vi "StageControl.vi"(9 "Stage Serial Number":i32=94839332, 11 "MG17Motor":refnum<k7>(container)) -> (0 "error IO":errorcluster, 3 "reference out":refnum<k7>)   [LabVIEW 2012]
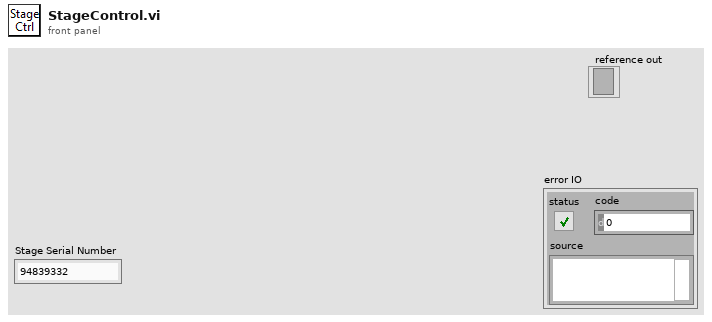
[diagram p1: front panel]
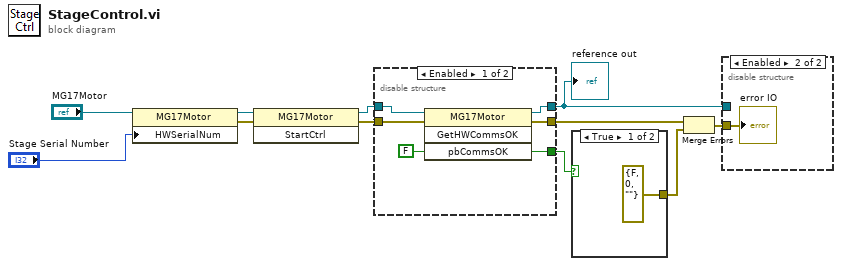
[diagram p0: block diagram]
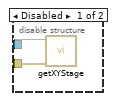
[diagram p2: hidden frame]
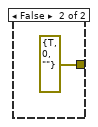
[diagram p4: hidden frame]
diagram:
  n1 = property class="MG17Motor"(reference="MG17Motor", "HWSerialNum"="Stage Serial Number") -> (reference out=w9:refnum<k7>, error out=w5:errorcluster)  [unwired: 1 in]
  n2 = invoke class="MG17Motor" method="StartCtrl"(reference=w9, error in=w5) -> (reference out=w11:refnum<k7>, error out=w10:errorcluster)  [unwired: 1 in, 1 out]
  n3 = disable-structure shown="Enabled" {
    disable-tunnel: w11 -> [w17 w19]
    disable-tunnel: w10 -> [w16 w18]
    disable-tunnel: [w14 _] -> w8
    disable-tunnel: [w13 w18] -> w7
    disable-tunnel: [w12 w19] -> w4
    frame Enabled {
      n4 = invoke class="MG17Motor" method="GetHWCommsOK"(reference=w17, error in=w16, "pbCommsOK"=FALSE) -> (reference out=w12:refnum<k7>, error out=w13:errorcluster, "pbCommsOK"=w14:bool)  [unwired: 1 in, 1 out]
    }
    frame Disabled {
    }
  }
  "reference out" <- w4
  n5 = case shown="True" w8 {
    tunnel: [errorcluster {"status"=FALSE, "code"=0, "source"=""} ("error in (no error)") errorcluster {"status"=TRUE, "code"=0, "source"=""} ("error in (no error)")] -> w6
    frame True {
    }
    frame False {
    }
  }
  n6 = Merge Errors(w7, w6) -> (w1:errorcluster)
  n7 = disable-structure shown="Enabled" {
    disable-tunnel: w4 -> [w23 _]
    disable-tunnel: w1 -> [w22 w24]
    frame Disabled {
      n8 = call "getXYStage.vi"("error in (no error)"=w22, "Thorlabs APT Stage In"=w23) -> ()  [unwired: 9 in, 1 out]
    }
    frame Enabled {
      "error IO" <- w24
    }
  }
